vi "Next.vi"(10 "error in (no error)":errorcluster, 11 "SequenceCountService in":refnum<class "SequenceCountService.lvclass">) -> (2 "error out":errorcluster, 3 "Sequence":u32)   [LabVIEW 2020, in "Vecto.lvlib" / "SequenceCountService.lvclass"]
uses:
  SequenceCountService.lvclass
  SequenceCountService.lvclass/SequenceCountService.ctl
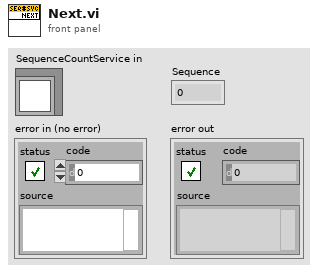
[diagram p1: front panel]
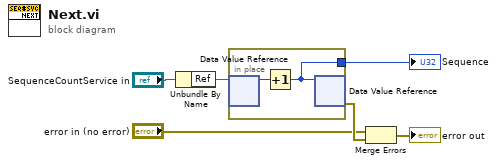
[diagram p0: block diagram]
diagram:
  n1 = Unbundle By Name("SequenceCountService in") -> ("Ref"=w6:refnum<data-value>)
  n2 = in-place {
    in-place-border: [w7] -> w4
    n3 = in-place-dvr #1(w6) -> (w8:u32)  [unwired: 1 out]
    n4 = Increment(x=w8) -> (x+1=w7:u32)
    n5 = in-place-dvr #1(w7) -> (w3:errorcluster)  [unwired: 1 out]
  }
  "Sequence" <- w4
  n6 = Merge Errors("error in (no error)", w3) -> (→"error out":errorcluster)
